vi "GP.vi"(8 "error in (no error)":errorcluster, 9 "Pin":u8, 10 "Puerto":u8, 11 "Serial Devices in":refnum<class "Serial Devices.lvclass">) -> (0 "error out":errorcluster, 3 "Serial Devices out":refnum<class "Serial Devices.lvclass">)   [LabVIEW 2019, in "Serial Devices.lvlib" / "Serial Devices.lvclass"]
uses:
  Serial Devices.lvclass
  C:/Program Files (x86)/National Instruments/LabVIEW 2019/vi.lib/ActorFramework/Actor/Actor.lvclass
  Serial Devices.lvclass/Serial Devices.ctl
  <vilib>/ActorFramework/Actor/Actor.lvclass/Actor.ctl
  <vilib>/ActorFramework/Message Enqueuer/Message Enqueuer.lvclass/Message Enqueuer.ctl
  NXP/NXP.lvclass
  TI/CYPRESS.lvclass
  SIMULATED/SIMULATED.lvclass
  <vilib>/ActorFramework/Message Enqueuer/Init from Existing Queue.vi
  <vilib>/ActorFramework/Message Enqueuer/Message Enqueuer.lvclass
  <vilib>/ActorFramework/Actor/Actor.lvclass
  Serial Devices.lvlib
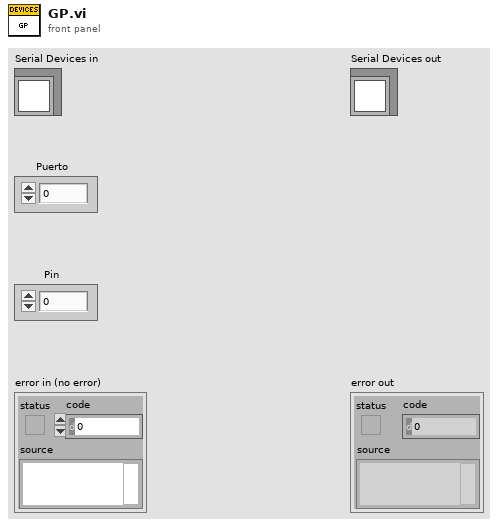
[diagram p1: front panel]
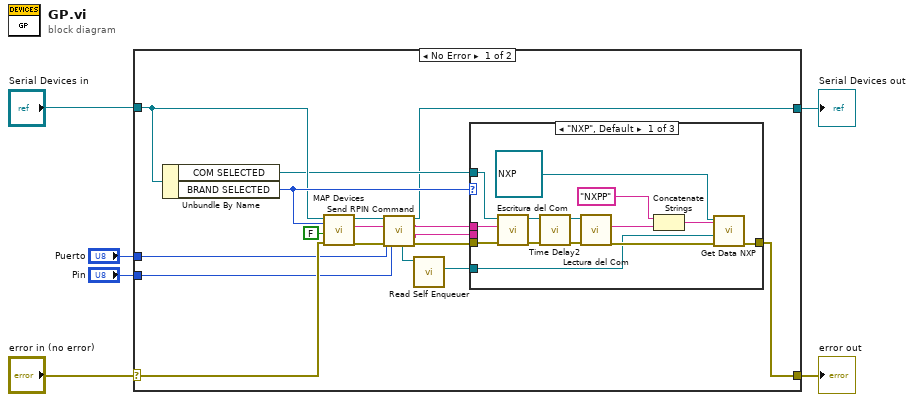
[diagram p0: block diagram]
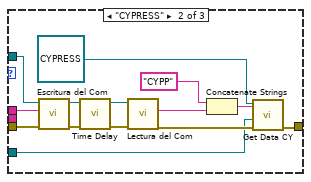
[diagram p2: hidden frame]
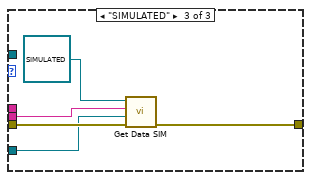
[diagram p3: hidden frame]
diagram:
  n1 = case shown="No Error" "error in (no error)" {
    selector: "error in (no error)" -> [w21 w55]
    tunnel: [w18 w55] -> w5
    tunnel: [w10 w54] -> w3
    tunnel: "Serial Devices in" -> [w17 w54]
    tunnel: "Puerto" -> [w8 _]
    tunnel: "Pin" -> [w9 _]
    frame No Error {
      n2 = Unbundle By Name(w17) -> ("COM SELECTED"=w16:refnum<visa-resource-name>, "BRAND SELECTED"=w20:enum16{"NXP", "CYPRESS", "SIMULATED"})
      n3 = call "MAP Devices.vi"("error in (no error)"=w21, "CREAR"=FALSE, "BRAND SELECTED"=w20, "Serial Devices in"=w17) -> ("error out"=w14:errorcluster, "VALOR"=w7:string, "Serial Devices out"=w15:refnum<class "Serial Devices.lvclass">)  [unwired: 5 in]
      n4 = call-dynamic "Send RPIN Command.vi"("Serial Devices in"=w15, "Device"=w7, "Puerto"=w8, "Pin"=w9, "error in"=w14) -> ("Serial Devices out"=w10:refnum<class "Serial Devices.lvclass">, "Command"=w11:string, "Expected"=w12:string, "error out"=w13:errorcluster)  [unwired: 7 in]
      n5 = call <vilib>:"Read Self Enqueuer.vi"("Actor"=w15) -> ("Self Enqueuer"=w19:refnum<class "Message Enqueuer.lvclass">)  [unwired: 10 in]
      n6 = case shown="\"NXP\", Default" w20 {
        tunnel: w13 -> [w35 w48 w52]
        tunnel: w12 -> [_ _ w51]
        tunnel: w19 -> [w28 w41 w50]
        tunnel: [w27 w40 w49] -> w18
        tunnel: w16 -> [w33 w47 _]
        tunnel: w11 -> [w34 w46 _]
        frame "NXP", Default {
          n7 = call "Escritura del Com.vi"("error in (no error)"=w35, "write buffer"=w34, "VISA Refnum in"=w33) -> ("error out"=w24:errorcluster, "VISA resource name out"=w32:refnum<visa-resource-name>)  [unwired: 7 in]
          n8 = call "Time Delay2"("error in (no error)"=w24) -> ("error out"=w23:errorcluster)  [unwired: 10 in]
          n9 = call "Lectura del Com.vi"("error in (no error)"=w23, "VISA Refnum in"=w32) -> ("error out"=w29:errorcluster, "Serial Response"=w30:string)  [unwired: 7 in, 1 out]
          n10 = Concatenate Strings("NXPP" ("string"), w30) -> (w26:string)
          n11 = call "Get Data NXP.vi"("error in"=w29, "Data Enqueuer"=w28, "Data"=w26, "NXP in"=refnum<class "NXP.lvclass"> refnum ("NXP.lvclass")) -> ("error out"=w27:errorcluster)  [unwired: 6 in, 1 out]
        }
        frame "CYPRESS" {
          n12 = call "Escritura del Com.vi"("error in (no error)"=w48, "write buffer"=w46, "VISA Refnum in"=w47) -> ("error out"=w36:errorcluster, "VISA resource name out"=w45:refnum<visa-resource-name>)  [unwired: 7 in]
          n13 = call "Time Delay"("error in (no error)"=w36) -> ("error out"=w37:errorcluster)  [unwired: 10 in]
          n14 = call "Lectura del Com.vi"("error in (no error)"=w37, "VISA Refnum in"=w45) -> ("error out"=w42:errorcluster, "Serial Response"=w43:string)  [unwired: 7 in, 1 out]
          n15 = Concatenate Strings("CYPP" ("string"), w43) -> (w39:string)
          n16 = call "Get Data CY.vi"("error in"=w42, "Data Enqueuer"=w41, "Data"=w39, "CYPRESS in"=refnum<class "CYPRESS.lvclass"> refnum ("CYPRESS.lvclass")) -> ("error out"=w40:errorcluster)  [unwired: 6 in, 1 out]
        }
        frame "SIMULATED" {
          n17 = call "Get Data SIM.vi"("error in"=w52, "Data Enqueuer"=w50, "Data"=w51, "SIMULATED in"=refnum<class "SIMULATED.lvclass"> refnum ("SIMULATED.lvclass")) -> ("error out"=w49:errorcluster)  [unwired: 6 in, 1 out]
        }
      }
    }
    frame Error {
    }
  }
  "error out" <- w5
  "Serial Devices out" <- w3
